vi "Save Files.vi"(8 "Error In":errorcluster, 9 "Relative Wiki Path":string="learn:libraries:linx:reference:labview", 10 "VI Data":T1, 11 "Output Root Directory":path=path "C:/Users/samkristoff/Desktop/Comment Test.vi") -> (0 "Error Out":errorcluster)   [LabVIEW 2014]
uses:
  VI Data.ctl
  Control Info.ctl
  <vilib>/picture/picture.llb/imagedata.ctl
  <vilib>/MakerHub/Toolbox/LMH-Toolbox.lvlib
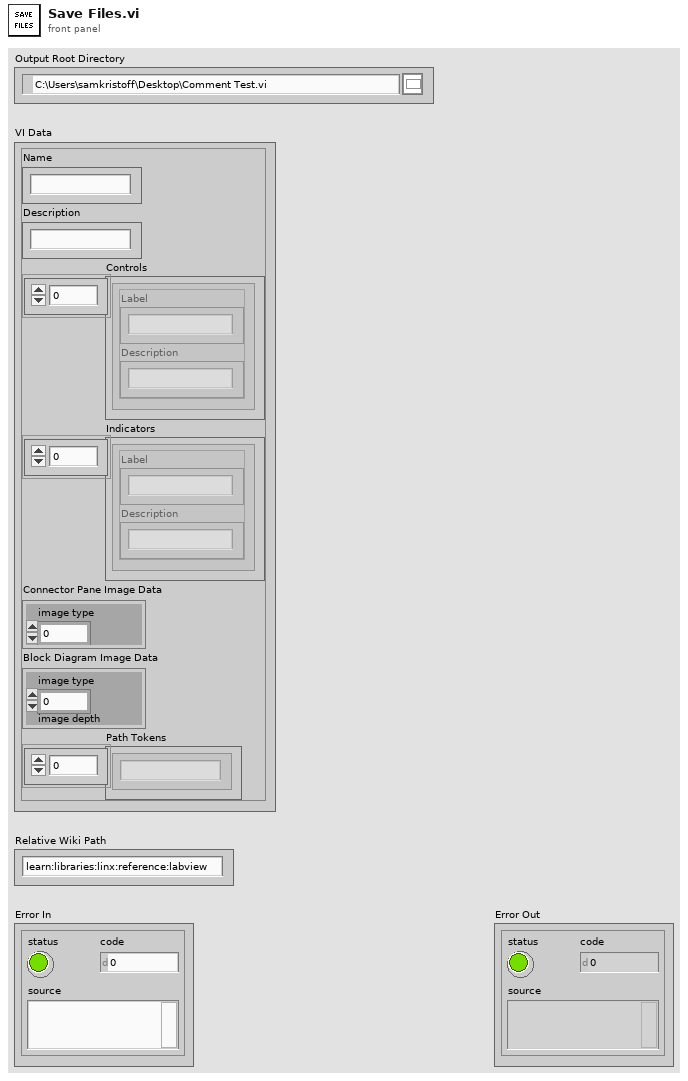
[diagram p1: front panel]
types:
  T1 = typedef "VI Data.ctl" = cluster{"Name":string, "Description":string, "Controls":T2[], "Indicators":T2[], "Connector Pane Image Data":T3, "Block Diagram Image Data":T3, "Path Tokens":string[]}
  T2 = typedef "Control Info.ctl" = cluster{"Label":string, "Description":string}
  T3 = typedef "imagedata.ctl" = cluster{"image type":i32, "image depth":i32, "image":u8[], "mask":u8[], "colors":u32[], "Rectangle":cluster{"left":i16, "top":i16, "right":i16, "bottom":i16}}
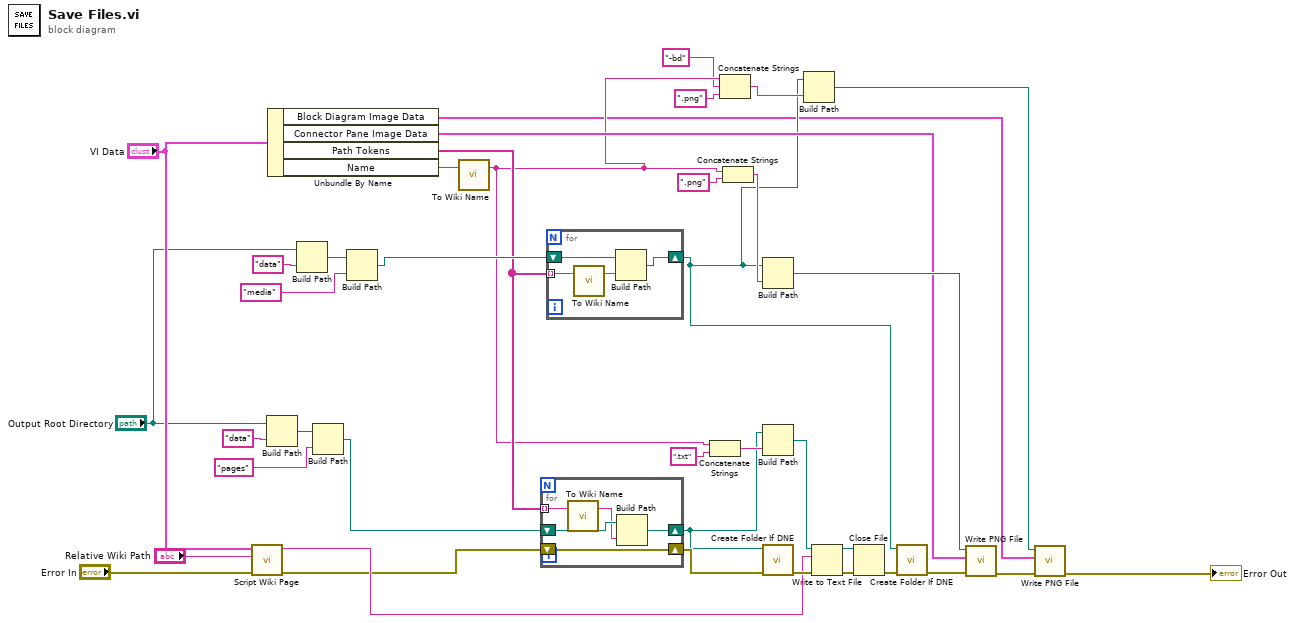
[diagram p0: block diagram]
diagram:
  n1 = call "Script Wiki Page.vi"("Error In"="Error In", "Relative Wiki Path"="Relative Wiki Path", "VI Data"="VI Data") -> ("Error Out"=w27:errorcluster, "Wiki Page Syntax"=w32:string)  [unwired: 7 in]
  n2 = Build Path(base path="Output Root Directory", name or relative path="data") -> (appended path=w22:path)
  n3 = Unbundle By Name("VI Data") -> ("Block Diagram Image Data"=w2:T3, "Connector Pane Image Data"=w26:T3, "Path Tokens"=w12:string[], "Name"=w11:string)
  n4 = Build Path(base path="Output Root Directory", name or relative path="data") -> (appended path=w21:path)
  n5 = Build Path(base path=w22, name or relative path="pages") -> (appended path=w15:path)
  n6 = Build Path(base path=w21, name or relative path="media") -> (appended path=w13:path)
  n7 = call "To Wiki Name.vi"("Name"=w11) -> ("Wiki Name"=w9:string)  [unwired: 2 in]
  n8 = for {
    shift-right: [w43] -> w14
    shift-left: w15 -> [w44]
    tunnel: w12 -> [w42] mode=indexing
    shift-right: [w40] -> w39
    shift-left: w27 -> [w40]
    n9 = call "To Wiki Name.vi"("Name"=w42) -> ("Wiki Name"=w41:string)  [unwired: 2 in]
    n10 = Build Path(base path=w44, name or relative path=w41) -> (appended path=w43:path)
  }
  n11 = for {
    shift-right: [w47] -> w4
    shift-left: w13 -> [w48]
    tunnel: w12 -> [w45] mode=indexing
    n12 = call "To Wiki Name.vi"("Name"=w45) -> ("Wiki Name"=w46:string)  [unwired: 2 in]
    n13 = Build Path(base path=w48, name or relative path=w46) -> (appended path=w47:path)
  }
  n14 = Concatenate Strings(w9, ".txt" ("string")) -> (w30:string)
  n15 = Concatenate Strings(w9, "-bd" ("Wiki Name"), ".png" ("string")) -> (w5:string)
  n16 = Concatenate Strings(w9, ".png" ("string")) -> (w37:string)
  n17 = Build Path(base path=w4, name or relative path=w37) -> (appended path=w38:path)
  n18 = Build Path(base path=w14, name or relative path=w30) -> (appended path=w31:path)
  n19 = call <vilib>:"Create Folder If DNE.vi"("Error In"=w39, "Folder Path"=w14) -> ("Error Out"=w35:errorcluster)  [unwired: 8 in, 1 out]
  n20 = Build Path(base path=w4, name or relative path=w5) -> (appended path=w3:path)
  n21 = Write to Text File(file (use dialog)=w31, text=w32, error in=w35) -> (refnum out=w34:refnum<file>, error out=w33:errorcluster)  [unwired: 1 in, 1 out]
  n22 = Close File(refnum=w34, error in=w33) -> (error out=w18:errorcluster)  [unwired: 1 out]
  n23 = call <vilib>:"Create Folder If DNE.vi"("Error In"=w18, "Folder Path"=w4) -> ("Error Out"=w17:errorcluster)  [unwired: 8 in, 1 out]
  n24 = call <vilib>:"Write PNG File.vi"("error in (no error)"=w17, "image data"=w26, "path to PNG file"=w38) -> ("error out"=w7:errorcluster)  [unwired: 7 in, 1 out]
  n25 = call <vilib>:"Write PNG File.vi"("error in (no error)"=w7, "image data"=w2, "path to PNG file"=w3) -> ("error out"=→"Error Out":errorcluster)  [unwired: 7 in, 1 out]
